vi ".NET Data Type Information to G Data Type Information.vi"(8 "error in (no error)":errorcluster, 9 ".NET Data Type Information":refnum<k24>, 11 "TwinCAT ADS in":refnum<class "TwinCAT ADS.lvclass">) -> (0 "error out":errorcluster, 2 "Data Type Information":T1 {"Category" items=["Unknown, None"=0, "Primitive"=1, "Alias"=2, "Enum"=3, "Array"=4, "Struct"=5, "FunctionBlock"=6, "Program"=7, "Function"=8, "SubRange"=9, "String"=10, "Bitset"=12, "Pointer"=13, "Union"=14, "Reference"=15, "Interface"=16]; "Type ID" items=["ADST_VOID"=0, "ADST_INT16"=2, "ADST_INT32"=3, "ADST_REAL32"=4, "ADST_REAL64"=5, "ADST_INT8"=16, "ADST_UINT8"=17, "ADST_UINT16"=18, "ADST_UINT32"=19, "ADST_INT64"=20, "ADST_UINT64"=21, "ADST_STRING"=30, "ADST_WSTRING"=31, "ADST_REAL80"=32, "ADST_BIT"=33, "ADST_MAXTYPES"=34, "ADST_BIGTYPE"=65]}, 3 "TwinCAT ADS out":refnum<class "TwinCAT ADS.lvclass">)   [LabVIEW 2018, in "TwinCAT ADS.lvclass"]
uses:
  TwinCAT ADS.lvclass
  TwinCAT.Ads
  Controls/Data Type Information.ctl
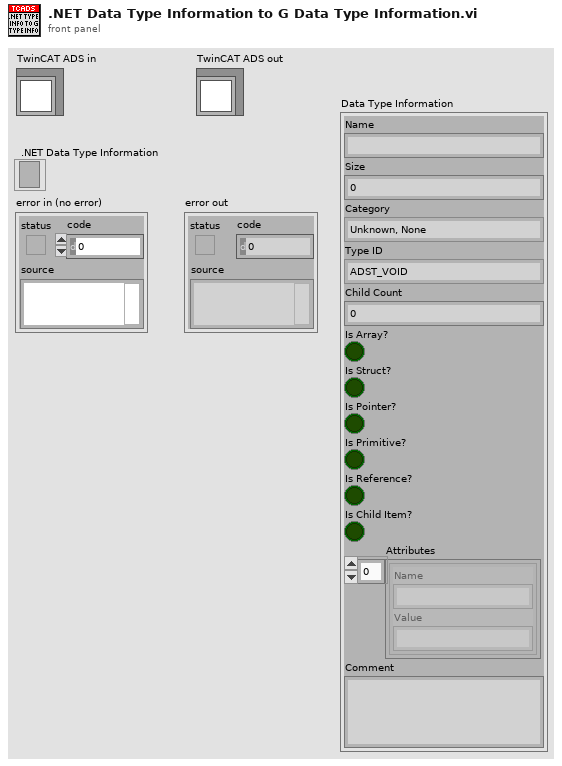
[diagram p1: front panel]
types:
  T1 = typedef "TwinCAT ADS.lvclass/Data Type Information.ctl" = cluster{"Name":string, "Size":i32, "Category":i32, "Type ID":i32, "Child Count":i32, "Is Array?":bool, "Is Struct?":bool, "Is Pointer?":bool, "Is Primitive?":bool, "Is Reference?":bool, "Is Child Item?":bool, "Attributes":cluster{"Name":string, "Value":string}[], "Comment":string}
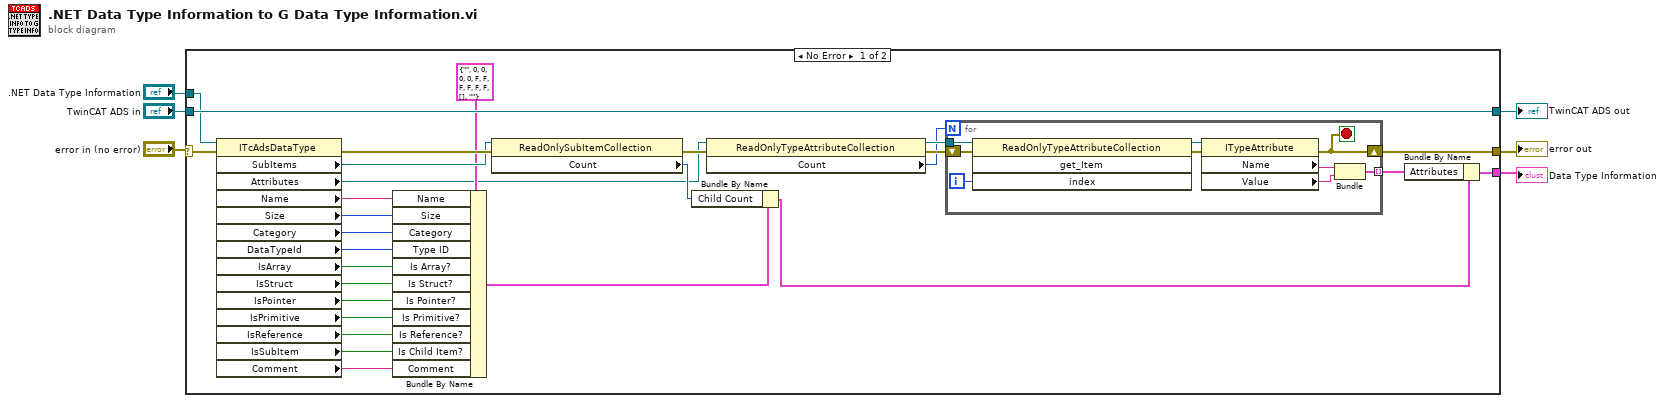
[diagram p0: block diagram]
diagram:
  n1 = case shown="No Error" "error in (no error)" {
    selector: "error in (no error)" -> [w33 w45]
    tunnel: [w16 w45] -> w5
    tunnel: [w34 w44] -> w3
    tunnel: "TwinCAT ADS in" -> [w34 w44]
    tunnel: ".NET Data Type Information" -> [w32 _]
    tunnel: [w17 _] -> w1
    frame No Error {
      n2 = property class="ITcAdsDataType"(reference=w32, error in=w33) -> (error out=w14:errorcluster, "SubItems"=w10:refnum<k24>, "Attributes"=w7:refnum<k24>, "Name"=w31:string, "Size"=w30:i32, "Category"=w29:i32, "DataTypeId"=w28:i32, "IsArray"=w15:bool, "IsStruct"=w27:bool, "IsPointer"=w26:bool, "IsPrimitive"=w25:bool, "IsReference"=w24:bool, "IsSubItem"=w23:bool, "Comment"=w22:string)  [unwired: 1 out]
      n3 = Bundle By Name(cluster=T1 {"Name"="", "Size"=0, "Category"=0, "Type ID"=0, "Child Count"=0, "Is Array?"=FALSE, "Is Struct?"=FALSE, "Is Pointer?"=FALSE, "Is Primitive?"=FALSE, "Is Reference?"=FALSE, "Is Child Item?"=FALSE, "Attributes"=[], "Comment"=""} ("Data Type Information"), "Name"=w31, "Size"=w30, "Category"=w29, "Type ID"=w28, "Is Array?"=w15, "Is Struct?"=w27, "Is Pointer?"=w26, "Is Primitive?"=w25, "Is Reference?"=w24, "Is Child Item?"=w23, "Comment"=w22) -> (w13:T1)
      n4 = property class="ReadOnlySubItemCollection"(reference=w10, error in=w14) -> (error out=w8:errorcluster, "Count"=w12:i32)  [unwired: 1 out]
      n5 = Bundle By Name(cluster=w13, "Child Count"=w12) -> (w11:T1)
      n6 = property class="ReadOnlyTypeAttributeCollection"(reference=w7, error in=w8) -> (reference out=w20:refnum<k24>, error out=w21:errorcluster, "Count"=w19:i32)
      n7 = for {
        N: w19 -> [_]
        tunnel: w20 -> [w43]
        tunnel: [w37] -> w18 mode=indexing
        shift-right: [w35] -> w16
        shift-left: w21 -> [w36]
        i -> [w42]
        stop <- w35 stop-if-true
        n8 = invoke class="ReadOnlyTypeAttributeCollection" method="get_Item"(reference=w43, error in=w36, "index"=w42) -> (error out=w41:errorcluster, "get_Item"=w40:refnum<k24>)  [unwired: 1 in, 2 out]
        n9 = property class="ITypeAttribute"(reference=w40, error in=w41) -> (error out=w35:errorcluster, "Name"=w39:string, "Value"=w38:string)  [unwired: 1 out]
        n10 = Bundle("Name"=w39, "Value"=w38) -> (w37:cluster{"Name":string, "Value":string})  [unwired: 1 in]
      }
      n11 = Bundle By Name(cluster=w11, "Attributes"=w18) -> (w17:T1)
    }
    frame Error {
    }
  }
  "error out" <- w5
  "TwinCAT ADS out" <- w3
  "Data Type Information" <- w1
